vi "RSS - Mouse.vi"(9 "Click":bool, 10 "y":i32, 11 "x":i32) -> ()   [LabVIEW 2020]
uses:
  user32.dll
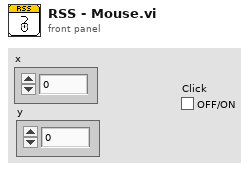
[diagram p1: front panel]
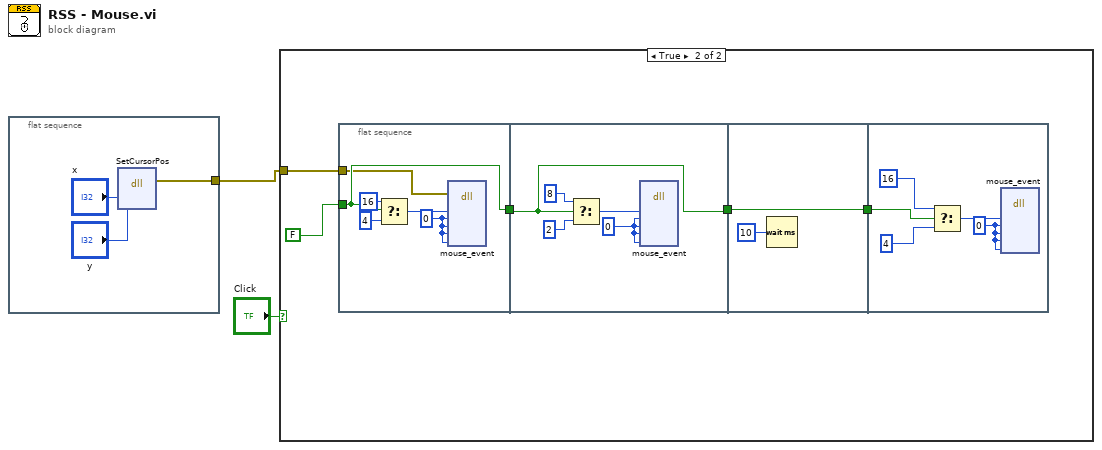
[diagram p0: block diagram]
diagram:
  n1 = flat-sequence {
    tunnel: [w3] -> w2
    frame #0 {
      n2 = dll-call lib="User32.dll" fn="SetCursorPos"("x"="x", "y"="y") -> (error out=w3:errorcluster)  [unwired: 3 in, 4 out]
    }
  }
  n3 = case shown="True" "Click" {
    tunnel: w2 -> [_ w6]
    frame False {
    }
    frame True {
      n4 = flat-sequence {
        tunnel: [w12] -> w10
        tunnel: FALSE -> [w12]
        tunnel: w6 -> [w11]
        tunnel: w10 -> [w21]
        tunnel: [w21] -> w9
        tunnel: w9 -> [w22]
        tunnel: [w22] -> w8
        tunnel: w8 -> [w28]
        frame #0 {
          w13 = 0 ("dx")
          n5 = Select(t=u32 16, s=w12, f=u32 4) -> (s? t:f=w16:u32)
          n6 = dll-call lib="User32.dll" fn="mouse_event"(error in=w11, "dwFlags"=w16, "dx"=w13, "dy"=w13, "dwData"=w13, "dwExtraInfo"=w13) -> ()  [unwired: 7 in, 3 out]
        }
        frame #1 {
          w20 = 0 ("dx")
          n7 = Select(t=u32 8, s=w21, f=u32 2) -> (s? t:f=w17:u32)
          n8 = dll-call lib="User32.dll" fn="mouse_event"("dwFlags"=w17, "dx"=w20, "dy"=w20, "dwData"=w20, "dwExtraInfo"=w20) -> ()  [unwired: 8 in, 3 out]
        }
        frame #2 {
          n9 = Wait (ms)(milliseconds to wait=u32 10) -> ()  [unwired: 1 out]
        }
        frame #3 {
          w27 = 0 ("dx")
          n10 = Select(t=u32 16, s=w28, f=u32 4) -> (s? t:f=w24:u32)
          n11 = dll-call lib="User32.dll" fn="mouse_event"("dwFlags"=w24, "dx"=w27, "dy"=w27, "dwData"=w27, "dwExtraInfo"=w27) -> ()  [unwired: 8 in, 3 out]
        }
      }
    }
  }
